vi "Ctrl-Visibility.vi"(0 "Quick-GUI-Update in":refnum<class "Quick-GUI-Update.lvclass">, 2 "Ctrl-Label":string[](array[string]), 11 "error in (no error)":errorcluster, 13 "Visibility":i32=3) -> (4 "Quick-GUI-Update out":refnum<class "Quick-GUI-Update.lvclass">, 15 "error out":errorcluster)   [LabVIEW 2020, in "Quick-GUI-Update.lvclass"]
doc: "<b>Visibility</b>\n1---><b>Show</b> Control's based on the given <b>Ctrl-Label</b> input.\n2---><b>Hide</b> Controls based ont he given <b>Ctrl-Label</b> input.\n3---><b>Show all</b> the control's in the Front Panel."
uses:
  Quick-GUI-Update.lvclass
  Quick-GUI-Update.lvclass/Quick-GUI-Update.ctl
  Ctrl Reference's/Ctrl Reference's.lvclass
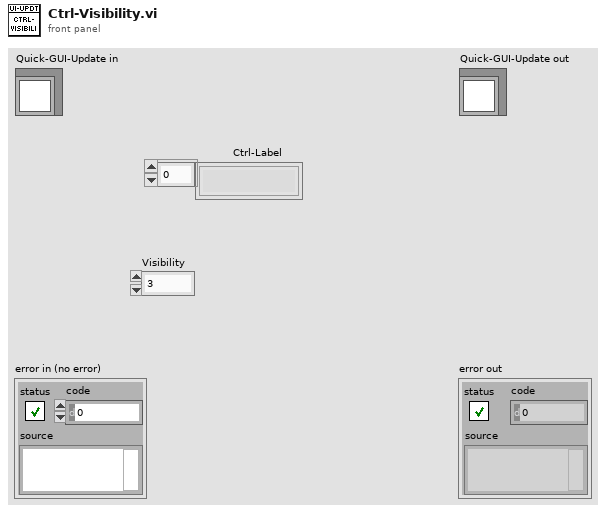
[diagram p1: front panel]
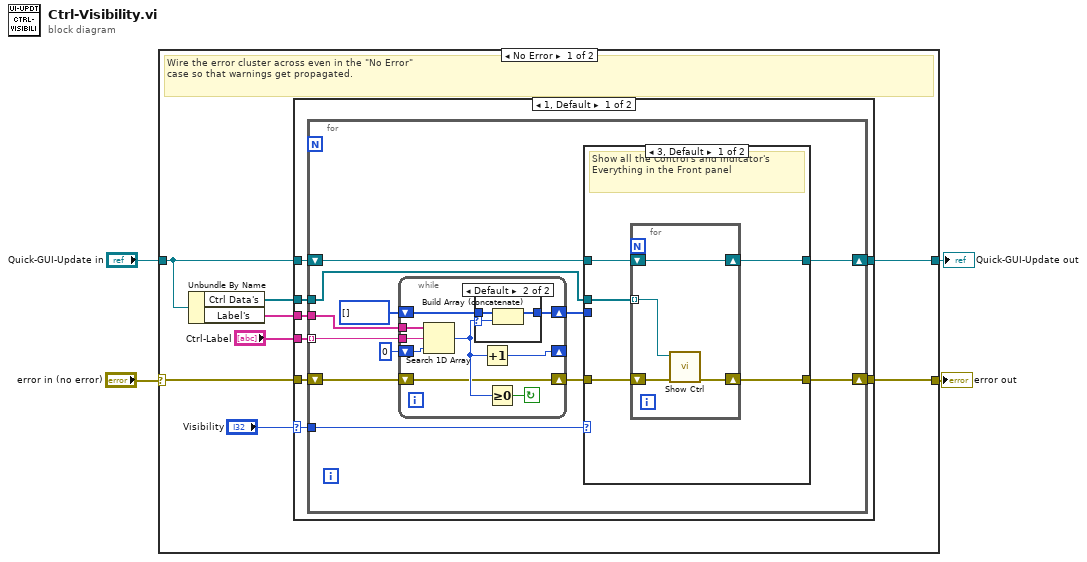
[diagram p0: block diagram]
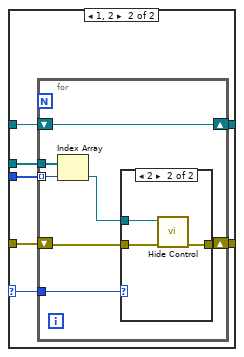
[diagram p3: hidden frame]
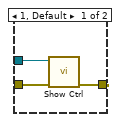
[diagram p4: hidden frame]
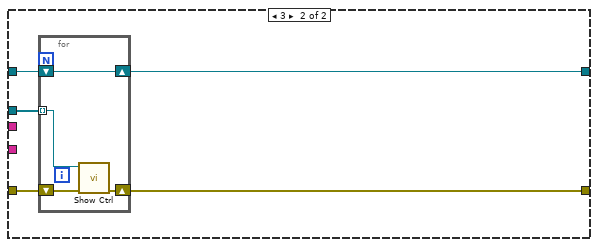
[diagram p5: hidden frame]
diagram:
  n1 = case shown="No Error" "error in (no error)" {
    selector: "error in (no error)" -> [w8 w85]
    tunnel: [w5 w85] -> w3
    tunnel: [w6 w84] -> w1
    tunnel: "Quick-GUI-Update in" -> [w7 w84]
    frame No Error {
      # "Wire the error cluster across even in the \"No Error\"\ncase so that warnings get propagated."
      n2 = Unbundle By Name(w7) -> ("Ctrl Data's"=w10:refnum<class "Ctrl Reference's.lvclass">[], "Label's"=w12:string[])
      n3 = case shown="1, Default" "Visibility" {
        selector: "Visibility" -> [w17 _]
        tunnel: w12 -> [w20 _]
        tunnel: "Ctrl-Label" -> [w19 _]
        tunnel: w10 -> [w18 w79]
        tunnel: w8 -> [w16 w78]
        tunnel: w7 -> [w15 w77]
        tunnel: [w14 w76] -> w6
        tunnel: [w13 w75] -> w5
        frame 1, Default {
          n4 = for {
            tunnel: w20 -> [w26]
            tunnel: w19 -> [w25] mode=indexing
            tunnel: w18 -> [w32]
            tunnel: w17 -> [w30]
            shift-right: [w31] -> w13
            shift-left: w16 -> [w23]
            shift-right: [w21] -> w14
            shift-left: w15 -> [w22]
            n5 = while {
              shift-right: [w34] -> _
              shift-left: 0 ("Start Index (0)") -> [w41]
              shift-right: [w38] -> w27
              shift-left: i32[] [] ("Initial Elements") -> [w39]
              tunnel: w26 -> [w40]
              tunnel: w25 -> [w37]
              shift-right: [w33] -> w24
              shift-left: w23 -> [w33]
              stop <- w35 continue-if-true
              n6 = Search 1D Array(1D array=w40, element=w37, start index (0)=w41) -> (index of element=w36:i32)
              n7 = case shown="Default" w36 {
                selector: w36 -> [_ w45]
                tunnel: w39 -> [w42 w44]
                tunnel: [w42 w43] -> w38
                frame -1 {
                }
                frame Default {
                  n8 = Build Array (concatenate)(w44, w45) -> (w43:i32[])
                }
              }
              n9 = Increment(x=w36) -> (x+1=w34:i32)
              n10 = Greater Or Equal To 0?(x=w36) -> (x >= 0?=w35:bool)
            }
            n11 = case shown="3, Default" w30 {
              selector: w30 -> [_ w57]
              tunnel: w24 -> [w50 w61]
              tunnel: w27 -> [_ w60]
              tunnel: w32 -> [w49 w59]
              tunnel: [w48 w58] -> w31
              tunnel: w22 -> [w47 w56]
              tunnel: [w46 w55] -> w21
              frame 3, Default {
                # "Show all the Control's and Indicator's Everything in the Front panel"
                n12 = for {
                  shift-right: [w51] -> w48
                  shift-left: w50 -> [w52]
                  tunnel: w49 -> [w53] mode=indexing
                  shift-right: [w54] -> w46
                  shift-left: w47 -> [w54]
                  n13 = call "Show Ctrl.vi"("error in (no error)"=w52, "Ctrl Reference's in"=w53) -> ("error out"=w51:errorcluster)  [unwired: 8 in, 1 out]
                }
              }
              frame 1, 2 {
                n14 = for {
                  shift-right: [w64] -> w58
                  shift-left: w61 -> [w63]
                  tunnel: w60 -> [w68] mode=indexing
                  tunnel: w59 -> [w67]
                  tunnel: w57 -> [w66]
                  shift-right: [w65] -> w55
                  shift-left: w56 -> [w65]
                  n15 = Index Array(array=w67, index=w68) -> (element=w62:refnum<class "Ctrl Reference's.lvclass">)
                  n16 = case shown="2" w66 {
                    tunnel: [w69 w73] -> w64
                    tunnel: w63 -> [w70 w74]
                    tunnel: w62 -> [w71 w72]
                    frame 1, Default {
                      n17 = call "Show Ctrl.vi"("error in (no error)"=w70, "Ctrl Reference's in"=w71) -> ("error out"=w69:errorcluster)  [unwired: 8 in, 1 out]
                    }
                    frame 2 {
                      n18 = call "Hide Control.vi"("error in (no error)"=w74, "Ctrl Reference's in"=w72) -> ("error out"=w73:errorcluster)  [unwired: 8 in, 1 out]
                    }
                  }
                }
              }
            }
          }
        }
        frame 3 {
          n19 = for {
            tunnel: w79 -> [w83] mode=indexing
            shift-right: [w82] -> w75
            shift-left: w78 -> [w81]
            shift-right: [w80] -> w76
            shift-left: w77 -> [w80]
            n20 = call "Show Ctrl.vi"("error in (no error)"=w81, "Ctrl Reference's in"=w83) -> ("error out"=w82:errorcluster)  [unwired: 8 in, 1 out]
          }
        }
      }
    }
    frame Error {
    }
  }
  "error out" <- w3
  "Quick-GUI-Update out" <- w1
